vi "Init Module.vi"(8 "error in":errorcluster, 11 "Singleton Module Admin in":refnum<class "Delacor_lib_QMH_Module Admin.lvclass">) -> (0 "error out":errorcluster, 2 "Database Request Events":T1, 3 "Singleton Module Admin out":refnum<class "Delacor_lib_QMH_Module Admin.lvclass">)   [LabVIEW 2021, in "Database.lvlib"]
doc: "Initialize the module by creating Broadcast Events, Request Events, and synchronization rendezvous.\n_____\nBased on DQMH Project Template 6.1.0.94."
uses:
  Database.lvlib
  <vilib>/Delacor/Delacor QMH/Libraries/Module Admin_class/Delacor_lib_QMH_Module Admin.lvclass
  Request Events--cluster.ctl
  Stop Argument--cluster.ctl
  Show Panel Argument--cluster.ctl
  Hide Panel Argument--cluster.ctl
  Get Module Execution Status Argument--cluster.ctl
  Show Diagram Argument--cluster.ctl
  REQ Add User Argument--cluster.ctl
  Class/DB/Credential.ctl
  REQ Check Credential Argument--cluster.ctl
  REQ Check Credential (Reply Payload)--cluster.ctl
  REQ Delete User Argument--cluster.ctl
  REQ Update User Details Argument--cluster.ctl
  Class/DB/Update Credential.ctl
  REQ List Table Argument--cluster.ctl
  REQ List Table (Reply Payload)--cluster.ctl
  REQ Delete Table Data Argument--cluster.ctl
  REQ Save DB Record Data Argument--cluster.ctl
  REQ Save Test Data Argument--cluster.ctl
  REQ Load Test Data Argument--cluster.ctl
  REQ Load Test Data (Reply Payload)--cluster.ctl
  REQ Get Username Argument--cluster.ctl
  REQ Get Username (Reply Payload)--cluster.ctl
  REQ Close DB Ref Argument--cluster.ctl
  REQ Retry DB Argument--cluster.ctl
  REQ DB Setup Argument--cluster.ctl
  REQ DB Setup (Reply Payload)--cluster.ctl
  REQ Write Test Info Argument--cluster.ctl
  User Interface/Test Info.ctl
  User Interface/User Interface.lvlib
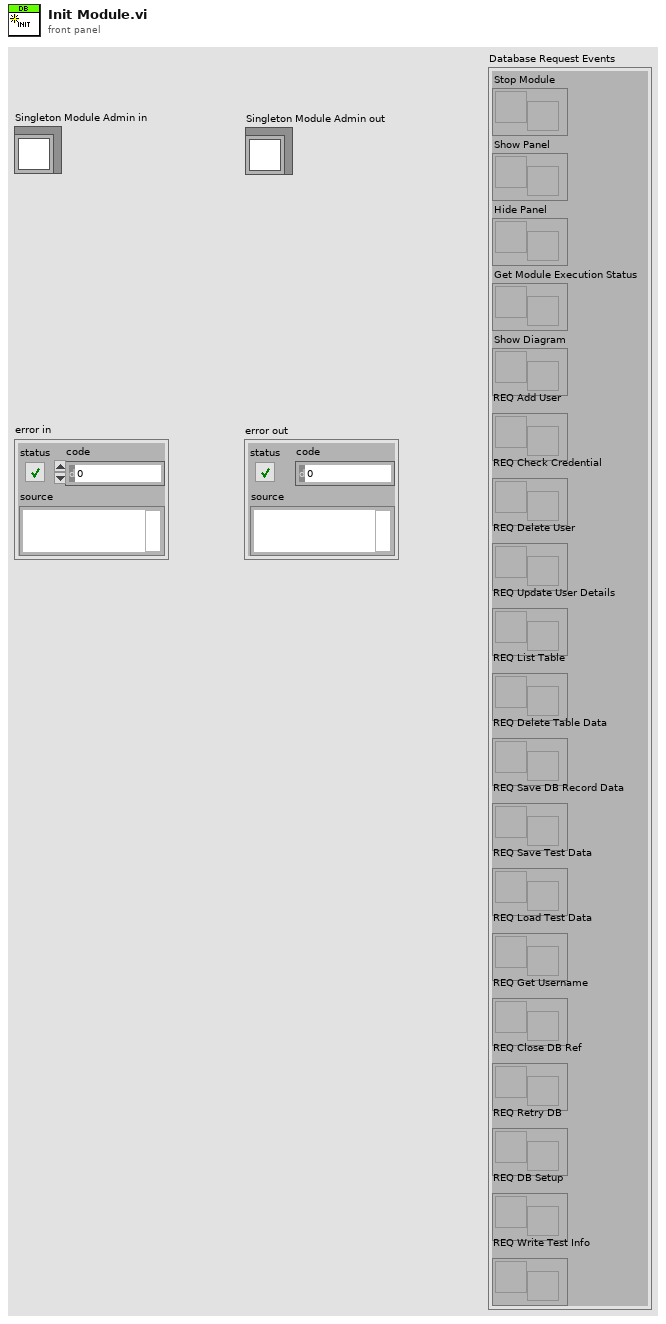
[diagram p1: front panel]
types:
  T1 = typedef "Database.lvlib/Request Events--cluster.ctl" = cluster{"Stop Module":refnum<user-event>, "Show Panel":refnum<user-event>, "Hide Panel":refnum<user-event>, "Get Module Execution Status":refnum<user-event>, "Show Diagram":refnum<user-event>, "REQ Add User":refnum<user-event>, "REQ Check Credential":refnum<user-event>, "REQ Delete User":refnum<user-event>, "REQ Update User Details":refnum<user-event>, "REQ List Table":refnum<user-event>, "REQ Delete Table Data":refnum<user-event>, "REQ Save DB Record Data":refnum<user-event>, "REQ Save Test Data":refnum<user-event>, "REQ Load Test Data":refnum<user-event>, "REQ Get Username":refnum<user-event>, "REQ Close DB Ref":refnum<user-event>, "REQ Retry DB":refnum<user-event>, "REQ DB Setup":refnum<user-event>, "REQ Write Test Info":refnum<user-event>}
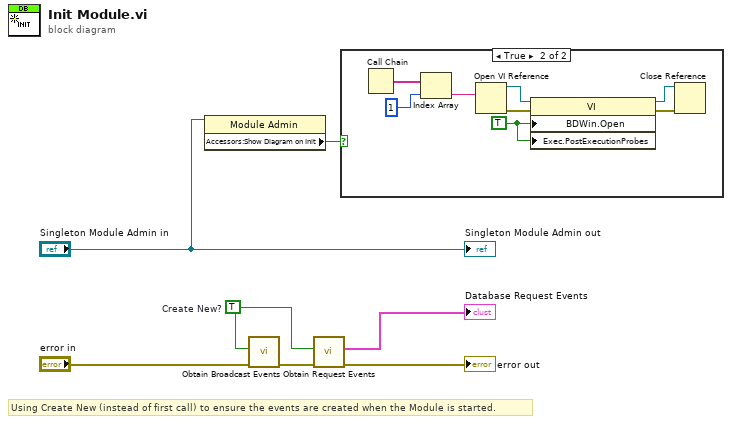
[diagram p0: block diagram]
diagram:
  w4 = TRUE  # Create New?
  # "Using Create New (instead of first call) to ensure the events are created when the Module is started."
  n1 = property class="Module Admin"(reference="Singleton Module Admin in") -> ("Accessors:Show Diagram on Init"=w2:bool)  [unwired: 1 in, 2 out]
  n2 = call "Obtain Broadcast Events.vi"("error in (no error)"="error in", "Create New? (F)"=w4) -> ("error out"=w7:errorcluster)  [unwired: 8 in, 1 out]
  n3 = call "Obtain Request Events.vi"("error in (no error)"=w7, "Create New? (F)"=w4) -> ("error out"=→"error out":errorcluster, "Database Request Events"=→"Database Request Events":T1)  [unwired: 8 in]
  n4 = case shown="True" w2 {
    frame False {
    }
    frame True {
      w11 = TRUE ("Block Diagram Window:Open")
      n5 = Call Chain() -> (call chain=w15:string[])
      n6 = Index Array(array=w15, index=1) -> (element=w8:string)
      n7 = Open VI Reference(vi path=w8) -> (vi reference=w12:refnum<vi>, error out=w13:errorcluster)  [unwired: 5 in]
      n8 = property class="VI"(reference=w12, error in=w13, "BDWin.Open"=w11, "Exec.PostExecutionProbes"=w11) -> (reference out=w9:refnum<vi>, error out=w10:errorcluster)
      n9 = Close Reference(reference=w9, error in (no error)=w10) -> ()  [unwired: 1 out]
    }
  }
  "Singleton Module Admin out" <- "Singleton Module Admin in"
